vi "Config Temperature.vi"(8 "error in (no error)":errorcluster, 11 "Configuration in":refnum<class "Configuration.lvclass">) -> (0 "error out":errorcluster, 3 "Configuration out":refnum<class "Configuration.lvclass">)   [LabVIEW 2016, in "Hardware.lvlib" / "VacuumLine.lvlib" / "VacuumLines Configuration.lvclass"]
uses:
  <userlib>/Common Components/Hardware/Abstract System/VacuumLine/VacuumLines Configuration/VacuumLines Configuration.lvclass
  <userlib>/Configuration Dialog Actor/Configuration.lvclass
  C:/Program Files (x86)/National Instruments/LabVIEW 2016/user.lib/Configuration Dialog Actor/Configuration.lvclass
panel:
  in  "Safe Temperature Range":cluster{"min":dbl, "max":dbl}={"min"=0.0, "max"=40.0}
  in  "Revert":bool
  in  "Apply":bool
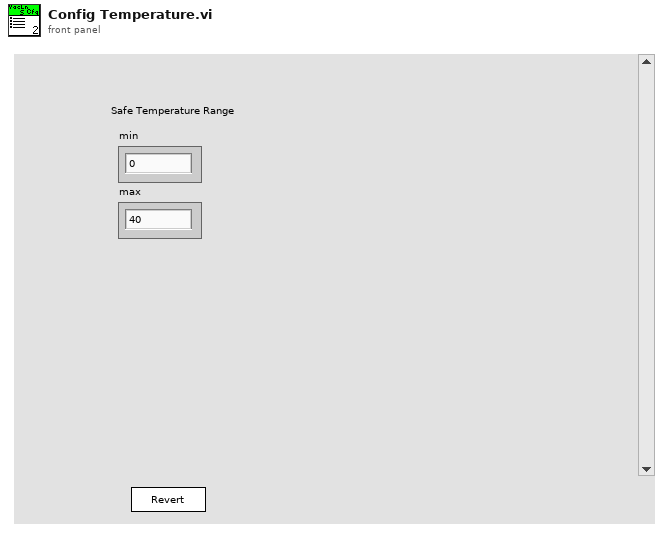
[diagram p1: front panel]
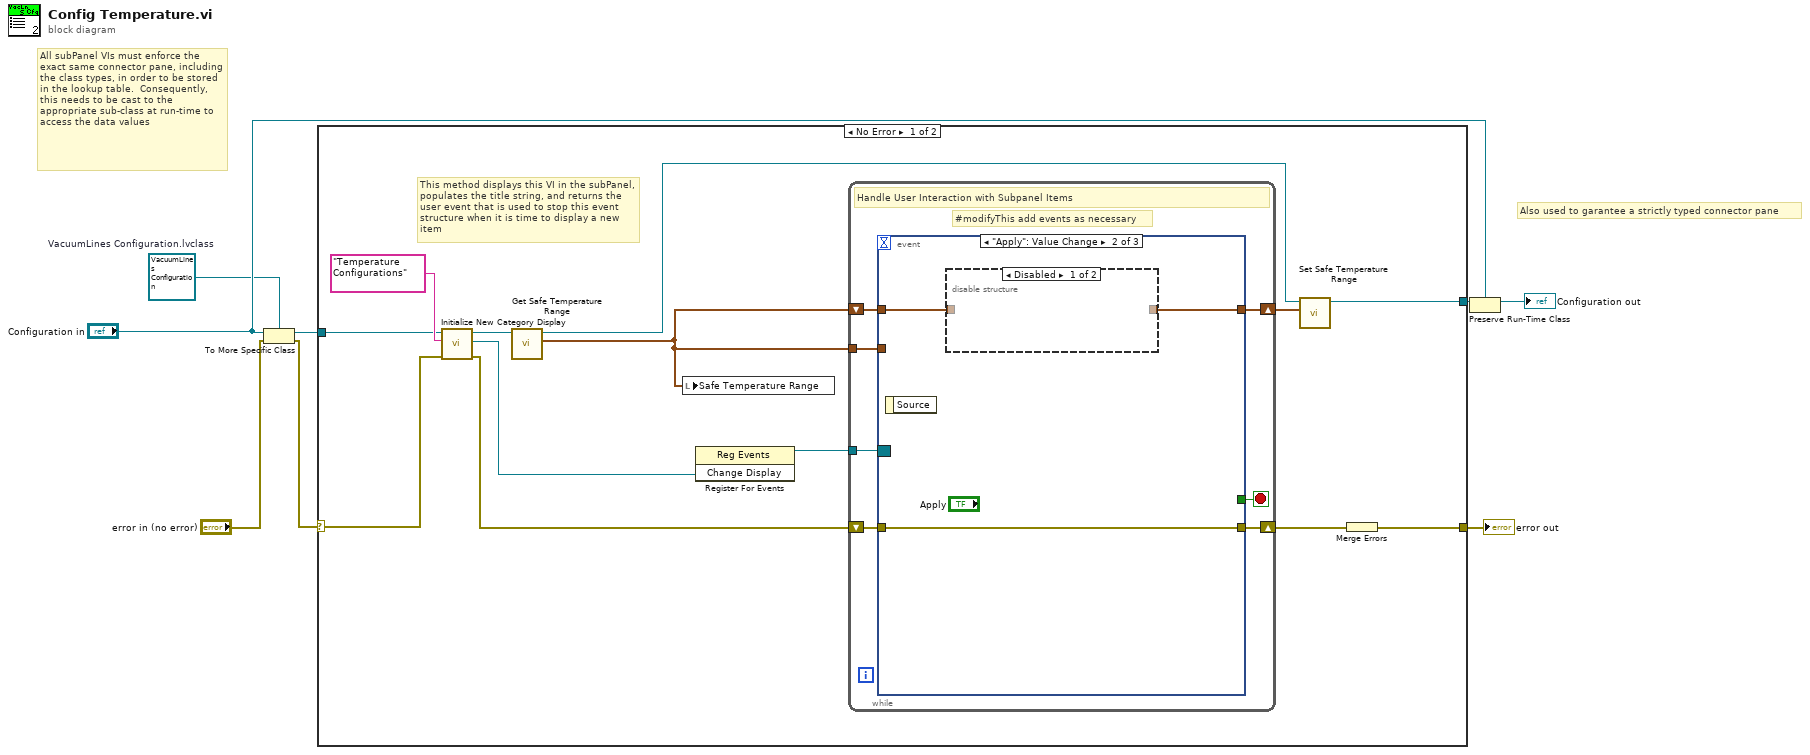
[diagram p0: block diagram]
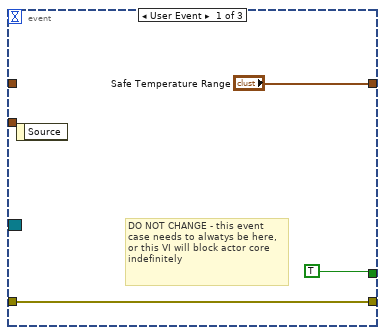
[diagram p2: hidden frame]
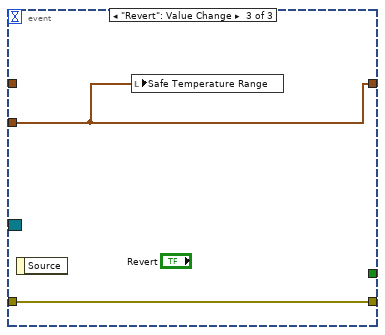
[diagram p4: hidden frame]
diagram:
  w2 = refnum<class "VacuumLines Configuration.lvclass"> refnum  # VacuumLines Configuration.lvclass
  # "Also used to garantee a strictly typed connector pane"
  # "All subPanel VIs must enforce the exact same connector pane, including the class types, in order to be stored in the lookup table.  Consequently, this needs to be cast to the appropriate sub-class at run-time to access the data values"
  n1 = To More Specific Class(target class=w2, reference="Configuration in", error in="error in (no error)") -> (specific class reference=w6:refnum<class "VacuumLines Configuration.lvclass">, error out=w1:errorcluster)
  n2 = case shown="No Error" w1 {
    selector: w1 -> [w15 w38]
    tunnel: w6 -> [w10 w39]
    tunnel: [w12 w39] -> w8
    tunnel: [w21 w38] -> w7
    frame No Error {
      # "This method displays this VI in the subPanel, populates the title string, and returns the user event that is used to stop this event structure when it is time to display a new item"
      n3 = call <userlib>:"Initialize New Category Display.vi"("error in (no error)"=w15, "Name to Display"="Temperature Configurations", "Configuration in"=w10) -> ("error out"=w16:errorcluster, "Change Display"=w19:refnum<user-event>, "Configuration Out"=w14:refnum<class "VacuumLines Configuration.lvclass">)  [unwired: 6 in]
      n4 = call <userlib>:"Get Safe Temperature Range.vi"("VacuumLines Configuration in"=w14) -> ("Safe Temperature Range"=w11:cluster{"min":dbl, "max":dbl}, "VacuumLines Configuration out"=w13:refnum<class "VacuumLines Configuration.lvclass">)  [unwired: 8 in, 1 out]
      n5 = local write "Safe Temperature Range"(w11) -> ()
      n6 = register-events(w19) -> (reference out=w18:refnum<event-registration>)  [unwired: 2 in, 1 out]
      n7 = while {
        tunnel: w18 -> [w27]
        shift-right: [w26] -> w17
        shift-left: w16 -> [w25]
        shift-right: [w23] -> w9
        shift-left: w11 -> [w24]
        tunnel: w11 -> [w22]
        stop <- w28 stop-if-true
        # "#modifyThis add events as necessary"
        # "Handle User Interaction with Subpanel Items"
        n8 = event shown="[1] \"Apply\": Value Change" {
          selector: w27 -> [_ _ _]
          dyn-events: _ -> [_ _ _]
          timeout: _ -> [_ _ _]
          tunnel: [TRUE _ _] -> w28
          tunnel: [w31 w34 w37] -> w26
          tunnel: w25 -> [w31 w34 w37]
          tunnel: w24 -> [_ w32 _]
          tunnel: ["Safe Temperature Range" w33 w36] -> w23
          tunnel: w22 -> [_ _ w36]
          event User Event {
            # "DO NOT CHANGE - this event case needs to alwatys be here, or this VI will block actor core indefinitely"
            n9 = event-data() -> ()  [unwired: 1 in, 1 out]
          }
          event "Apply": Value Change {
            n10 = event-data() -> ()  [unwired: 1 in, 1 out]
            n11 = disable-structure shown="Disabled" {
              disable-tunnel: [_ w35] -> w33
              disable-tunnel: w32 -> [_ w35]
              frame Disabled {
              }
              frame Enabled {
              }
            }
          }
          event "Revert": Value Change {
            n12 = event-data() -> ()  [unwired: 1 in, 1 out]
            n13 = local write "Safe Temperature Range"(w36) -> ()
          }
        }
      }
      n14 = call <userlib>:"Set Safe Temperature Range.vi"("Safe Temperature Range"=w9, "VacuumLines Configuration in"=w13) -> ("VacuumLines Configuration out"=w12:refnum<class "VacuumLines Configuration.lvclass">)  [unwired: 8 in, 1 out]
      n15 = Merge Errors(w17) -> (w21:errorcluster)
    }
    frame Error {
    }
  }
  "error out" <- w7
  n16 = Preserve Run-Time Class(object in=w8, 2:"Configuration in") -> (object out=→"Configuration out":refnum<class "Configuration.lvclass">)  [unwired: 1 in, 1 out]
